vi "Set NodeIDs.vi"(8 "error in (no error)":errorcluster, 9 "Deliminated Char":string=".", 10 "PLC Folder Names":string[](array[string]), 11 "OPC UA in":refnum<class "OPC UA.lvclass">) -> (0 "error out":errorcluster, 3 "OPC UA out":refnum<class "OPC UA.lvclass">)   [LabVIEW 2021, in "OPC UA.lvclass"]
uses:
  OPC UA.lvclass
  OPC UA.lvclass/OPC UA.ctl
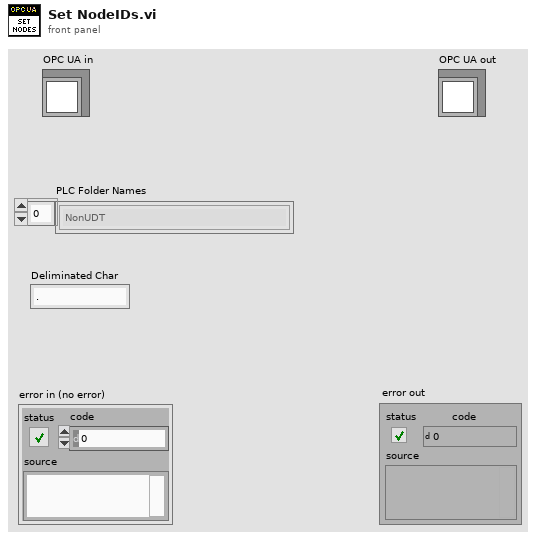
[diagram p1: front panel]
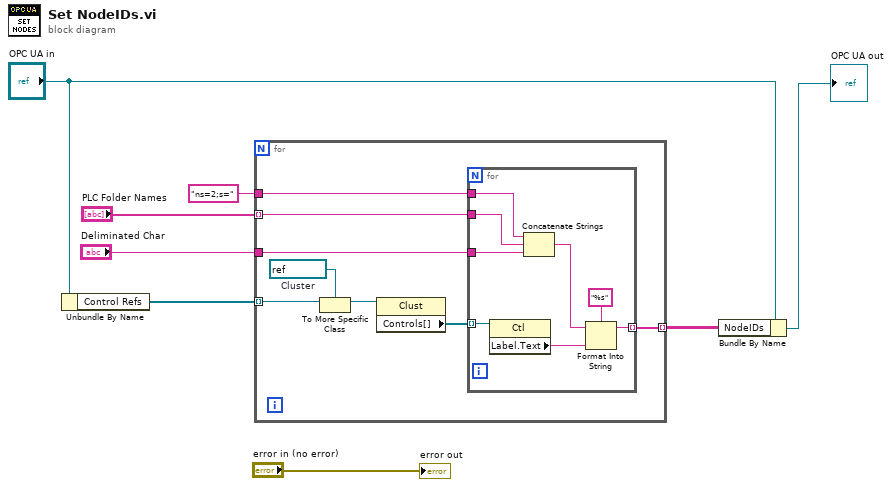
[diagram p0: block diagram]
diagram:
  n1 = Unbundle By Name("OPC UA in") -> ("Control Refs"=w3:refnum<vi>[])
  n2 = for {
    tunnel: "ns=2;s=" ("format string") -> [w16]
    tunnel: [w15] -> w6 mode=indexing
    tunnel: "PLC Folder Names" -> [w14] mode=indexing
    tunnel: w3 -> [w12] mode=indexing
    tunnel: "Deliminated Char" -> [w9]
    w11 = refnum<vi> refnum  # Cluster
    n3 = To More Specific Class(target class=w11, reference=w12) -> (specific class reference=w10:refnum<vi>)  [unwired: 1 in, 1 out]
    n4 = property class="Clust"(reference=w10) -> ("Controls[]"=w13:refnum<vi>[])  [unwired: 1 in, 2 out]
    n5 = for {
      tunnel: w13 -> [w24] mode=indexing
      tunnel: w14 -> [w20]
      tunnel: [w21] -> w15 mode=indexing
      tunnel: w16 -> [w19]
      tunnel: w9 -> [w17]
      n6 = property class="Ctl"(reference=w24) -> ("Label.Text"=w23:string)  [unwired: 1 in, 2 out]
      n7 = Concatenate Strings(w19, w20, w17) -> (w18:string)
      n8 = Format Into String(format string="%s", initial string=w18, w23) -> (resulting string=w21:string)  [unwired: 1 in, 1 out]
    }
  }
  n9 = Bundle By Name(cluster="OPC UA in", "NodeIDs"=w6) -> (→"OPC UA out":refnum<class "OPC UA.lvclass">)
  "error out" <- "error in (no error)"
